vi "Bitparallele Ansteuerung.vi"   [LabVIEW 2020, in "Funktionstasten.lvlib"]
uses:
  Funktionstasten.lvlib
  Funktionstasten-Aktion.ctl
  Zustaende.ctl
  cRIO/PC/Kommunikation mit cRIO.lvlib
types:
  T1 = typedef "Verwaltung - cRIO.lvlib/Digital Eingaenge 0-15.ctl" = cluster{"I0: N2 Nachf. FT-IR voll":bool, "I1: N2 Nachf. Vorrat leer":bool, "I2: (Klimaanlage eingeschaltet)":bool, "I3: (Klimaanlage Störung)":bool, "I4: Trigger Eingang (Messdaten sp.)":bool, "I5: Reserve":bool, "I6: Reserve":bool, "I7: Reserve":bool, "I8: Druckschalter Versorgung ok":bool, "I9: Reserve":bool, "I10: Reserve":bool, "I11: Reserve":bool, "I12: Drucksch. N2 Versorgung":bool, "I13: Reserve":bool, "I14: Reserve":bool, "I15: (Füllstand Kondensatbehälter)":bool}
  T2 = typedef "Funktionstasten.lvlib/Zustaende.ctl" = enum16{"Standby", "Pause", "Eco", "Messen", "Kalibrieren", "Spülen Filter", "Spülen Leitung", "Umgebungsluft", "0-Gas", "Cal-Gas", "CG zu PNS", "-------------", "Init 1", "Init 2", "Init 3", "Init 4", "Messen vorbereiten", "Messen durchführen", "Exit"}
  T3 = typedef "Funktionstasten.lvlib/Funktionstasten-Aktion.ctl" = enum16{"Initialisieren", "Zustand setzen", "Taste gedrückt", "Fehler speichern", "Lesen", "Manuell", "Remote", "Bitparallel", "Samplepoint", "Zeit Prüfen", "reset Umschalten"}
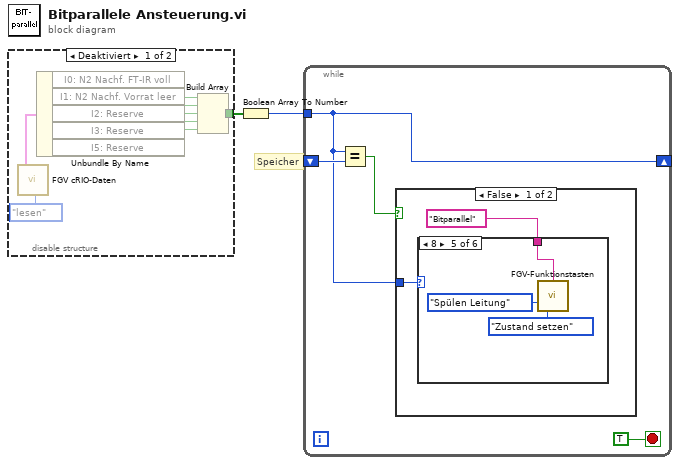
[diagram p0: block diagram]
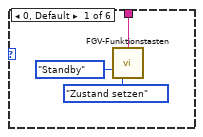
[diagram p3: hidden frame]
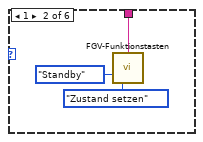
[diagram p4: hidden frame]
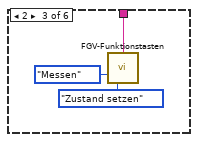
[diagram p5: hidden frame]
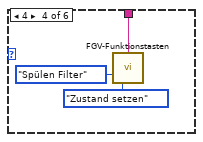
[diagram p6: hidden frame]
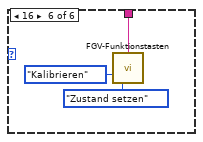
[diagram p7: hidden frame]
diagram:
  # "Speicher"
  n1 = disable-structure shown="Deaktiviert" {
    disable-tunnel: [w4 _] -> w2
    frame Disabled {
      n2 = call "FGV cRIO-Daten.vi"("Aktion"=enum16{"lesen", "schreiben"}."lesen") -> ("DI"=w10:T1)  [unwired: 9 in, 9 out]
      n3 = Unbundle By Name(w10) -> ("I0: N2 Nachf. FT-IR voll"=w9:bool, "I1: N2 Nachf. Vorrat leer"=w8:bool, "I2: Reserve"=w7:bool, "I3: Reserve"=w6:bool, "I5: Reserve"=w5:bool)
      n4 = Build Array(w9, w8, w7, w6, w5) -> (w4:bool[])
    }
    frame Enabled {
    }
  }
  n5 = Boolean Array To Number(Boolean array=w2) -> (number=w1:u32)
  n6 = while {
    shift-right: [w11] -> _
    shift-left: _ -> [w13]
    tunnel: w1 -> [w11]
    stop <- TRUE stop-if-true
    n7 = Equal?(x=w11, y=w13) -> (x = y?=w12:bool)
    n8 = case shown="False" w12 {
      tunnel: w11 -> [w16 _]
      frame False {
        n9 = case shown="8" w16 {
          tunnel: "Bitparallel" ("Herkunft") -> [w17 w20 w23 w26 w29 w32]
          frame 0, Default {
            n10 = call "FGV-Funktionstasten.vi"("Herkunft"=w17, "Zustand"=Zustaende."Standby", "Aktion"=Funktionstasten-Aktion."Zustand setzen") -> ()  [unwired: 5 in, 8 out]
          }
          frame 1 {
            n11 = call "FGV-Funktionstasten.vi"("Herkunft"=w20, "Zustand"=Zustaende."Standby", "Aktion"=Funktionstasten-Aktion."Zustand setzen") -> ()  [unwired: 5 in, 8 out]
          }
          frame 2 {
            n12 = call "FGV-Funktionstasten.vi"("Herkunft"=w23, "Zustand"=Zustaende."Messen", "Aktion"=Funktionstasten-Aktion."Zustand setzen") -> ()  [unwired: 5 in, 8 out]
          }
          frame 4 {
            n13 = call "FGV-Funktionstasten.vi"("Herkunft"=w26, "Zustand"=Zustaende."Spülen Filter", "Aktion"=Funktionstasten-Aktion."Zustand setzen") -> ()  [unwired: 5 in, 8 out]
          }
          frame 8 {
            n14 = call "FGV-Funktionstasten.vi"("Herkunft"=w29, "Zustand"=Zustaende."Spülen Leitung", "Aktion"=Funktionstasten-Aktion."Zustand setzen") -> ()  [unwired: 5 in, 8 out]
          }
          frame 16 {
            n15 = call "FGV-Funktionstasten.vi"("Herkunft"=w32, "Zustand"=Zustaende."Kalibrieren", "Aktion"=Funktionstasten-Aktion."Zustand setzen") -> ()  [unwired: 5 in, 8 out]
          }
        }
      }
      frame True {
      }
    }
  }
